vi "ReadTest (host).vi"() -> ()   [LabVIEW 2012]
uses:
  <vilib>/rvi/interface/nirviOpenFPGA/nirviOpenFPGA.xnode
  ReadTest (FPGA).vi
  <vilib>/rvi/interface/nirviReadWriteControl/nirviReadWriteControl.xnode
  <vilib>/rvi/interface/RandomDataEmulation/nirviRandomDataOpen.vi
panel:
  out "Points Read":i32
  out "Read uSec":u32
  in  "Stop":bool
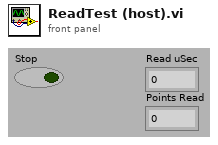
[diagram p1: front panel]
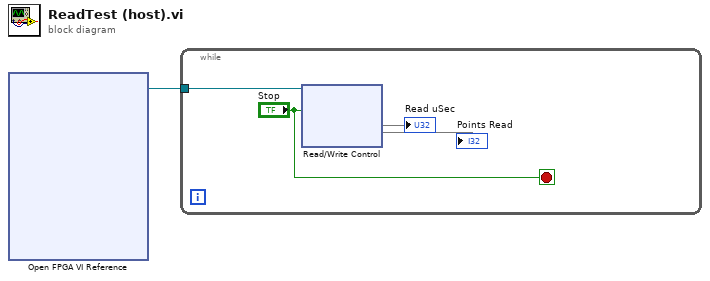
[diagram p0: block diagram]
diagram:
  n1 = xnode "Open FPGA VI Reference"() -> ("FPGA VI Reference Out"=w1:refnum<k20>)  [unwired: 2 in, 1 out]
  n2 = while {
    tunnel: w1 -> [w5]
    stop <- "Stop" stop-if-true
    n3 = xnode "Read/Write Control"("FPGA VI Reference In"=w5, "Stop"="Stop") -> ("Read uSec"=→"Read uSec", "Points Read"=→"Points Read")  [unwired: 1 in, 2 out]
  }
